vi "InterceptBallTactic_Init.vi"(0 "object in":refnum<class "InterceptBallTactic.lvclass">, 5 "error in (no error)":errorcluster) -> (14 "object out":refnum<class "InterceptBallTactic.lvclass">, 19 "error out":errorcluster)   [LabVIEW 2023, in "InterceptBallTactic.lvclass"]
uses:
  InterceptBallTactic.lvclass
  NewSTP/NewTactics/Tactic_v2_class/Tactic_v2.lvclass
  C:/Users/ebert/Documents/codes/SSL/repo/SSL_AI/NewSTP/NewTactics/Tactic_v2_class/Tactic_v2.lvclass
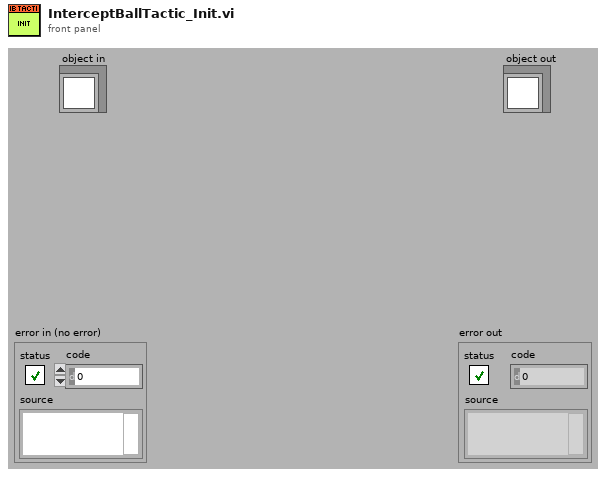
[diagram p1: front panel]
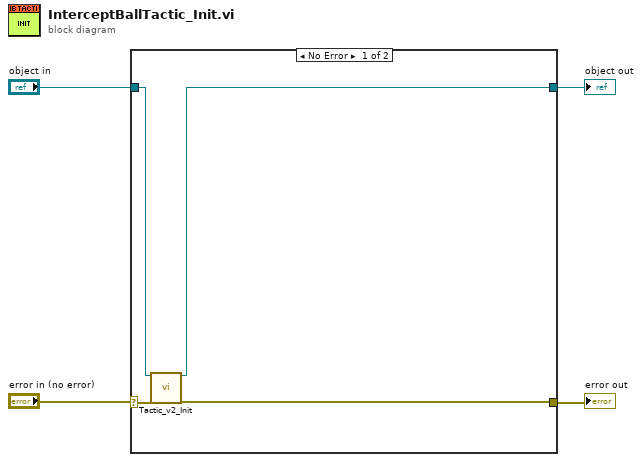
[diagram p0: block diagram]
diagram:
  n1 = case shown="No Error" "error in (no error)" {
    selector: "error in (no error)" -> [w7 w9]
    tunnel: "object in" -> [w8 w10]
    tunnel: [w5 w10] -> w3
    tunnel: [w6 w9] -> w1
    frame No Error {
      n2 = call "Tactic_v2_Init.vi"("object in"=w8, "error in (no error)"=w7) -> ("object out"=w5:refnum<class "InterceptBallTactic.lvclass">, "error out"=w6:errorcluster)  [unwired: 16 in]
    }
    frame Error {
    }
  }
  "object out" <- w3
  "error out" <- w1
